vi "PS Control Read v0.80.vi"(5 "error in (no error)":errorcluster) -> (0 "error out":errorcluster, 1 "Cell":string, 2 "Current":dbl caption="Current [kA]" format="%.5f", 3 "Status":T1, 4 "Time(ms)":u32)   [LabVIEW 2019]
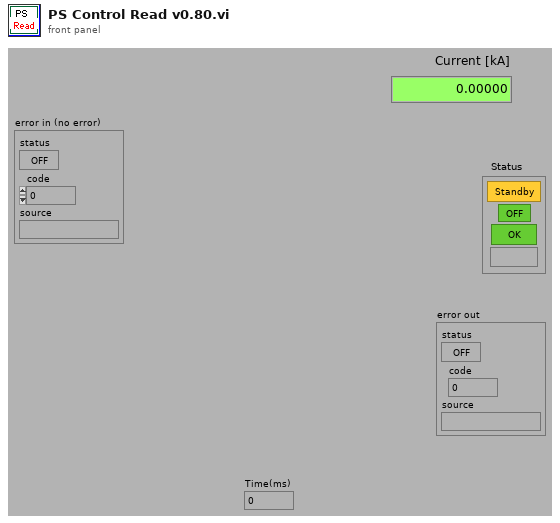
[diagram p1: front panel]
types:
  T1 = cluster{"PS on/off":bool, "PS fault?":bool, "Ramp Status":u16, "PS Control?":bool}
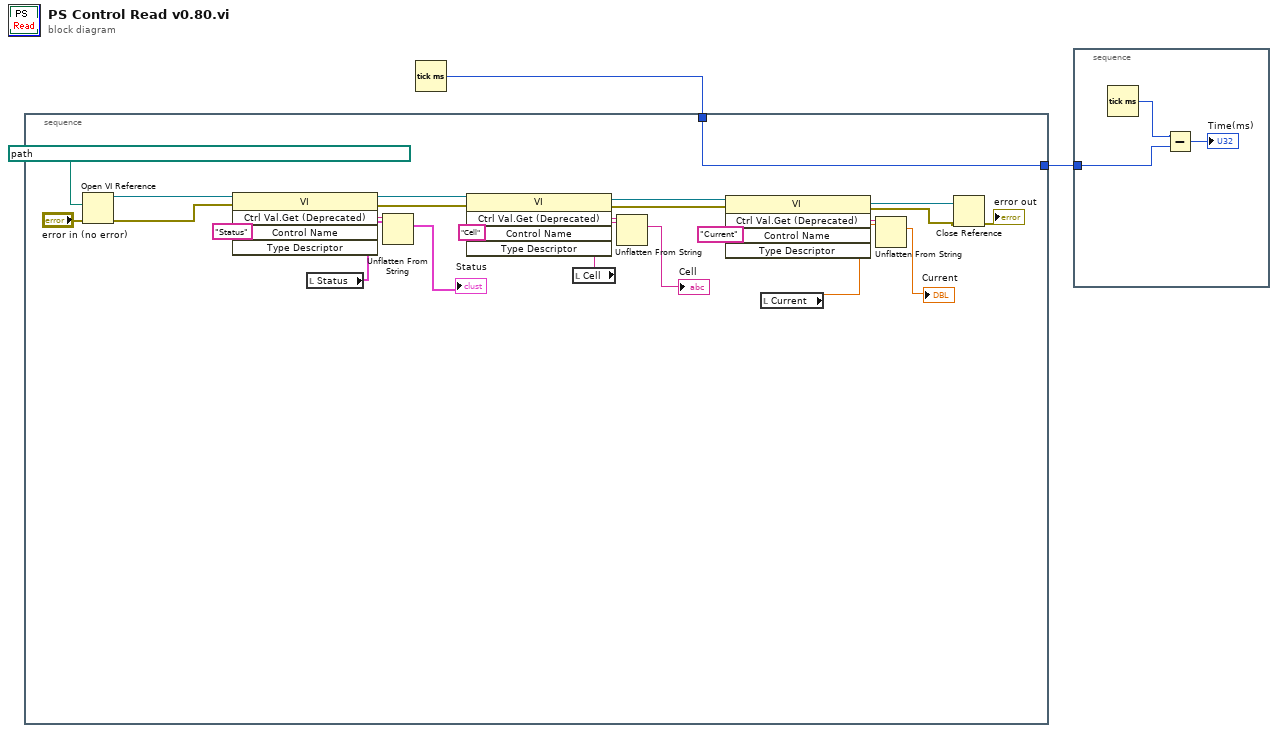
[diagram p0: block diagram]
diagram:
  n1 = Tick Count (ms)() -> (millisecond timer value=w2:u32)
  n2 = stacked-sequence {
    tunnel: [w13] -> w1
    tunnel: w2 -> [w13]
    frame #0 {
      n3 = Open VI Reference(vi path=path "/Optics2Mac/xwei Work/NML Data Acq/Serial Instruments/PS Ä/PS Control", error in (no error)="error in (no error)") -> (vi reference=w10:refnum<vi>, error out=w7:errorcluster)  [unwired: 4 in]
      n4 = invoke class="VI" method="Ctrl Val.Get (Deprecated)"(reference=w10, error in=w7, "Control Name"="Status") -> (reference out=w18:refnum<vi>, error out=w6:errorcluster, "Get Control Value"=w22:string)  [unwired: 2 in, 2 out]
      n5 = local read "Status"() -> (w19:T1)
      n6 = Unflatten From String(type=w19, binary string=w22) -> (value=→"Status":T1)  [unwired: 3 in, 2 out]
      n7 = invoke class="VI" method="Ctrl Val.Get (Deprecated)"(reference=w18, error in=w6, "Control Name"="Cell") -> (reference out=w14:refnum<vi>, error out=w5:errorcluster, "Get Control Value"=w24:string)  [unwired: 2 in, 2 out]
      n8 = local read "Cell"() -> (w17:string)
      n9 = Unflatten From String(type=w17, binary string=w24) -> (value=→"Cell":string)  [unwired: 3 in, 2 out]
      n10 = invoke class="VI" method="Ctrl Val.Get (Deprecated)"(reference=w14, error in=w5, "Control Name"="Current") -> (reference out=w11:refnum<vi>, error out=w4:errorcluster, "Get Control Value"=w20:string)  [unwired: 2 in, 2 out]
      n11 = local read "Current"() -> (w12:dbl)
      n12 = Unflatten From String(type=w12, binary string=w20) -> (value=→"Current":dbl)  [unwired: 3 in, 2 out]
      n13 = Close Reference(reference=w11, error in (no error)=w4) -> (error out=→"error out":errorcluster)
    }
  }
  n14 = stacked-sequence {
    tunnel: w1 -> [w28]
    frame #0 {
      n15 = Tick Count (ms)() -> (millisecond timer value=w29:u32)
      n16 = Subtract(x=w29, y=w28) -> (x-y=→"Time(ms)":u32)
    }
  }
